vi "Mess-Modus-ersetzen.vi"(1 "Eingangs-String":string) -> (0 "Ergebnis-String":string)   [LabVIEW 2019]
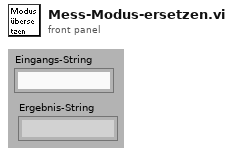
[diagram p1: front panel]
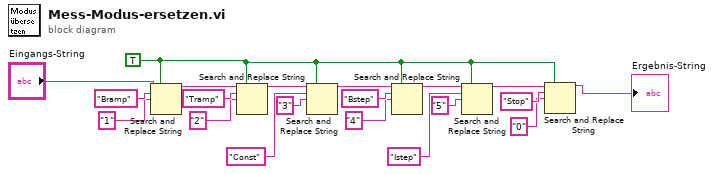
[diagram p0: block diagram]
diagram:
  w1 = TRUE ("Alle ersetzen? (F)")
  n1 = Search and Replace String(replace all?=w1, input string="Eingangs-String", search string="Bramp" ("Such-String"), replace string="1" ("String ersetzen(\"\")")) -> (result string=w10:string)  [unwired: 4 in, 3 out]
  n2 = Search and Replace String(replace all?=w1, input string=w10, search string="Tramp" ("Such-String"), replace string="2" ("String ersetzen(\"\")")) -> (result string=w9:string)  [unwired: 4 in, 3 out]
  n3 = Search and Replace String(replace all?=w1, input string=w9, search string="Const" ("Such-String"), replace string="3" ("String ersetzen(\"\")")) -> (result string=w8:string)  [unwired: 4 in, 3 out]
  n4 = Search and Replace String(replace all?=w1, input string=w8, search string="Bstep" ("Such-String"), replace string="4" ("String ersetzen(\"\")")) -> (result string=w7:string)  [unwired: 4 in, 3 out]
  n5 = Search and Replace String(replace all?=w1, input string=w7, search string="Istep" ("Such-String"), replace string="5" ("String ersetzen(\"\")")) -> (result string=w5:string)  [unwired: 4 in, 3 out]
  n6 = Search and Replace String(replace all?=w1, input string=w5, search string="Stop" ("String ersetzen(\"\")"), replace string="0" ("Such-String")) -> (result string=→"Ergebnis-String":string)  [unwired: 4 in, 3 out]
